vi "MSScript_Transform_UIntArray.vi"(5 "upper limit (18446744073709551615)":u64=18446744073709551615, 7 "lower limit (0)":u64, 8 "MinSize":i32=-1, 9 "MaxSize":i32=-1, 11 "Check_Str":string) -> (1 "Is a variable?":bool, 2 "Value Error?":bool, 3 "Value Output":u64[](array[numeric]))   [LabVIEW 2018, in "MSScript.lvclass"]
uses:
  MSScript.lvclass
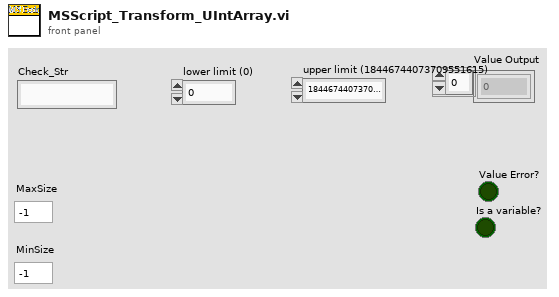
[diagram p1: front panel]
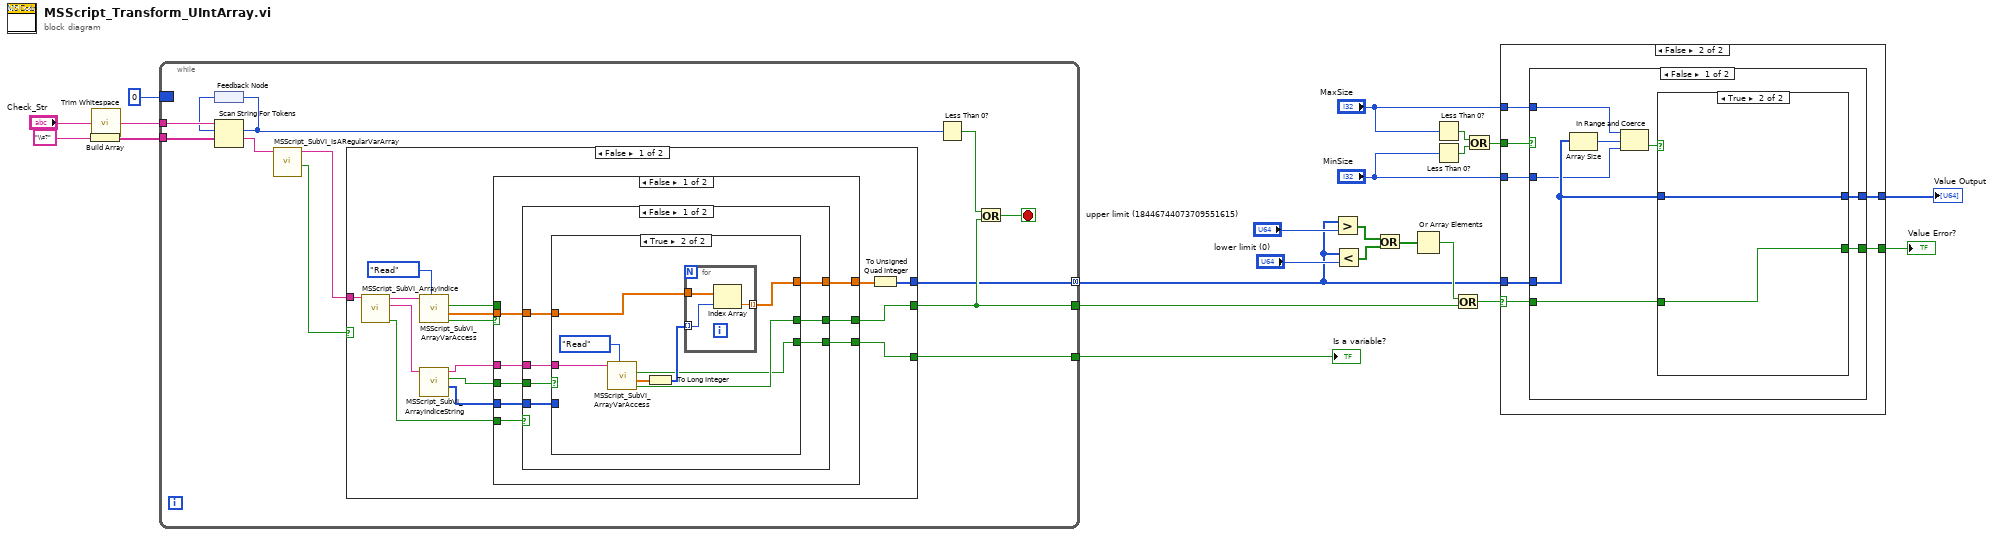
[diagram p0: block diagram]
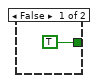
[diagram p3: hidden frame]
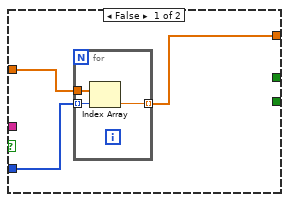
[diagram p5: hidden frame]
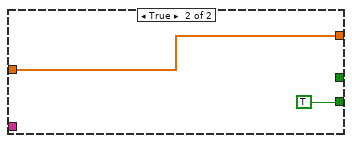
[diagram p6: hidden frame]
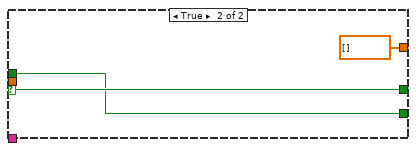
[diagram p7: hidden frame]
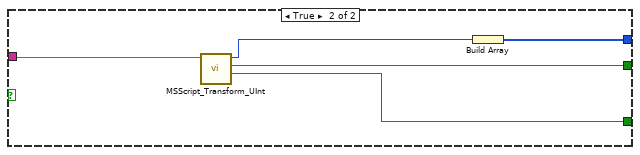
[diagram p8: hidden frame]
diagram:
  n1 = Build Array("\\s?" ("regular expression")) -> (w20:string[])
  n2 = call <vilib>:"Trim Whitespace.vi"("string"="Check_Str") -> ("trimmed string"=w10:string)  [unwired: 1 in]
  n3 = while {
    tunnel: w10 -> [w34]
    tunnel: w20 -> [w30]
    tunnel: [w23] -> w1 mode=concatenating
    tunnel: [w29] -> w12
    tunnel: [w24] -> w6
    border: 0 ("offset") -> [_]
    stop <- w25 stop-if-true
    n4 = feedback #1() -> (w33:i32)
    n5 = Scan String For Tokens(7:w30, 8:w33, 9:w34) -> (1:w28:string, 2:w32:i32)  [unwired: 3 in, 2 out]
    n6 = feedback-in #1(w32) -> ()
    n7 = call "MSScript_SubVI_IsARegularVarArray.vi"("VarString in"=w28) -> ("Variable simbol no found"=w26:bool, "VarString out"=w27:string)  [unwired: 6 in, 1 out]
    n8 = case shown="False" w26 {
      tunnel: [w35 w89] -> w23
      tunnel: [w45 w88] -> w24
      tunnel: [w38 w87] -> w29
      tunnel: w27 -> [w48 w91]
      frame False {
        n9 = call "MSScript_SubVI_ArrayIndice.vi"("@name[x:y|z]"=w48) -> ("Index no found"=w39:bool, "Indice string"=w43:string, "@name"=w47:string)  [unwired: 6 in]
        n10 = call "MSScript_SubVI_ArrayVarAccess.vi"("Function (Read)"=enum16{"Init", "Write", "Read"}."Read", "VarName"=w47) -> ("Value Error?"=w44:bool, "ArrayVariable out"=w46:ext[], "Is a variable ?"=w37:bool)  [unwired: 5 in]
        n11 = call "MSScript_SubVI_ArrayIndiceString.vi"("indice string in"=w43) -> ("x:y"=w40:i32[], "Indice string?"=w41:bool, "Array indice string out"=w42:string)  [unwired: 8 in]
        n12 = case shown="False" w44 {
          selector: w44 -> [_ w85]
          tunnel: w39 -> [w57 _]
          tunnel: [w56 ext[] [] ("ArrayVariable out")] -> w36
          tunnel: w46 -> [w55 _]
          tunnel: [w54 w85] -> w45
          tunnel: [w53 w84] -> w38
          tunnel: w41 -> [w52 _]
          tunnel: w40 -> [w51 _]
          tunnel: w42 -> [w50 _]
          tunnel: w37 -> [_ w84]
          frame False {
            n13 = case shown="False" w57 {
              tunnel: [w61 w83] -> w56
              tunnel: w55 -> [w62 w83]
              tunnel: [w59 _] -> w54
              tunnel: [w58 TRUE] -> w53
              tunnel: w52 -> [w64 _]
              tunnel: w51 -> [w63 _]
              tunnel: w50 -> [w60 _]
              frame False {
                n14 = case shown="True" w64 {
                  tunnel: w63 -> [w67 _]
                  tunnel: w62 -> [w66 w74]
                  tunnel: [w65 w73] -> w61
                  tunnel: w60 -> [_ w77]
                  tunnel: [_ w72] -> w59
                  tunnel: [_ w71] -> w58
                  frame False {
                    n15 = for {
                      tunnel: w67 -> [w70] mode=indexing
                      tunnel: w66 -> [w69]
                      tunnel: [w68] -> w65 mode=indexing
                      n16 = Index Array(array=w69, index=w70) -> (element=w68:ext)
                    }
                  }
                  frame True {
                    n17 = call "MSScript_SubVI_ArrayVarAccess.vi"("Function (Read)"=enum16{"Init", "Write", "Read"}."Read", "VarName"=w77) -> ("Value Error?"=w72:bool, "ArrayVariable out"=w76:ext[], "Is a variable ?"=w71:bool)  [unwired: 5 in]
                    n18 = To Long Integer(number=w76) -> (32bit integer=w75:i32[])
                    n19 = for {
                      tunnel: w75 -> [w81] mode=indexing
                      tunnel: w74 -> [w80]
                      tunnel: [w79] -> w73 mode=indexing
                      n20 = Index Array(array=w80, index=w81) -> (element=w79:ext)
                    }
                  }
                }
              }
              frame True {
              }
            }
          }
          frame True {
          }
        }
        n21 = To Unsigned Quad Integer(1:w36) -> (0:w35:u64[])
      }
      frame True {
        n22 = call "MSScript_Transform_UInt.vi"("string in"=w91) -> ("Is a variable ?"=w87:bool, "Value Error?"=w88:bool, "Value Output"=w90:u64)  [unwired: 8 in]
        n23 = Build Array(w90) -> (w89:u64[])
      }
    }
    n24 = Less Than 0?(x=w32) -> (x < 0?=w31:bool)
    n25 = Or(x=w31, y=w24) -> (x .or. y?=w25:bool)
  }
  "Is a variable?" <- w12
  n26 = Greater?(x=w1, y="upper limit (18446744073709551615)") -> (0:w9:bool[])
  n27 = Less?(x=w1, y="lower limit (0)") -> (x < y?=w8:bool[])
  n28 = Or(x=w9, y=w8) -> (x .or. y?=w7:bool[])
  n29 = Or Array Elements(Boolean array=w7) -> (logical OR=w5:bool)
  n30 = Less Than 0?(x="MaxSize") -> (x < 0?=w15:bool)
  n31 = Less Than 0?(x="MinSize") -> (x < 0?=w16:bool)
  n32 = Or(x=w5, y=w6) -> (x .or. y?=w4:bool)
  n33 = Or(x=w15, y=w16) -> (x .or. y?=w14:bool)
  n34 = case shown="False" w4 {
    selector: w4 -> [w92 w93]
    tunnel: w1 -> [_ w99]
    tunnel: [w92 w98] -> w19
    tunnel: "MaxSize" -> [_ w97]
    tunnel: "MinSize" -> [_ w96]
    tunnel: w14 -> [_ w95]
    tunnel: [_ w94] -> w13
    frame True {
    }
    frame False {
      n35 = case shown="False" w95 {
        tunnel: w99 -> [w106 w112]
        tunnel: [w104 w111] -> w98
        tunnel: w97 -> [w103 _]
        tunnel: w96 -> [w102 _]
        tunnel: [w101 w112] -> w94
        tunnel: w93 -> [w100 w111]
        frame False {
          n36 = Array Size(array=w106) -> (size(s)=w107:i32)
          n37 = In Range and Coerce(upper limit=w103, x=w107, lower limit=w102) -> (In Range?=w105:bool)  [unwired: 1 out]
          n38 = case shown="True" w105 {
            tunnel: w106 -> [_ w110]
            tunnel: [TRUE w109] -> w104
            tunnel: [_ w110] -> w101
            tunnel: w100 -> [_ w109]
            frame False {
            }
            frame True {
            }
          }
        }
        frame True {
        }
      }
    }
  }
  "Value Error?" <- w19
  "Value Output" <- w13
